vi "License Generator.vi"() -> ()   [LabVIEW 2015]
panel:
  in  "Day":i32
  out "deadline":timestamp
  out "current time":timestamp
  out "date/time string":string
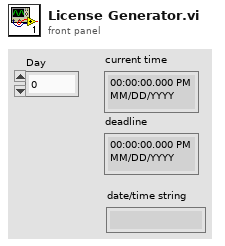
[diagram p1: front panel]
types:
  T1 = enum16{"open", "replace", "create", "open or create", "replace or create", "replace or create with confirmation"}
  T2 = cluster{"seconds since 1Jan1904":timestamp, timestamp}
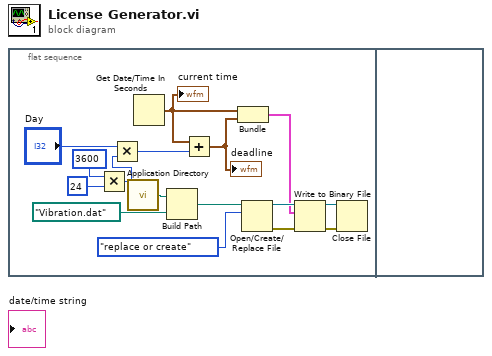
[diagram p0: block diagram]
diagram:
  n1 = flat-sequence {
    frame #0 {
      n2 = Multiply(x=3600, y=24) -> (x*y=w2:i32)
      n3 = Multiply(x="Day", y=w2) -> (x*y=w5:i32)
      n4 = call <vilib>:"Application Directory.vi"() -> ("Application Directory"=w15:path)
      n5 = Get Date/Time In Seconds() -> (seconds since 1Jan1904=w9:timestamp)
      "current time" <- w9
      n6 = Build Path(base path=w15, name or relative path=path "Vibration.dat") -> (appended path=w6:path)
      n7 = Add(x=w9, y=w5) -> (x+y=w8:timestamp)
      "deadline" <- w8
      n8 = Bundle("seconds since 1Jan1904"=w9, w8) -> (w7:T2)  [unwired: 1 in]
      n9 = Open/Create/Replace File(file path (use dialog)=w6, operation (0:open)=T1."replace or create") -> (refnum out=w13:refnum<file>, error out=w12:errorcluster)  [unwired: 4 in, 1 out]
      n10 = Write to Binary File(file (use dialog)=w13, data=w7, error in=w12) -> (refnum out=w10:refnum<file>, error out=w11:errorcluster)  [unwired: 3 in, 1 out]
      n11 = Close File(refnum=w10, error in=w11) -> ()  [unwired: 2 out]
    }
    frame #1 {
    }
  }
